vi "GetCurPageFromTabCtrl.vi"(11 "tab ctrl in":refnum<vi>) -> (2 "값":variant, 3 "tab ctrl out":refnum<vi>)   [LabVIEW 2018, in "Library-Ctrl.lvlib"]
uses:
  Library-Ctrl.lvlib
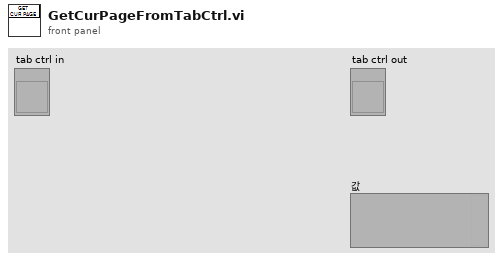
[diagram p1: front panel]
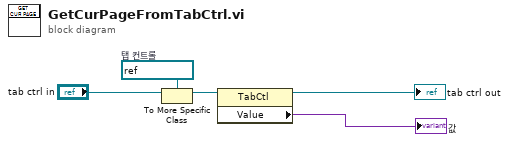
[diagram p0: block diagram]
diagram:
  w4 = refnum<vi> refnum  # 탭 컨트롤
  n1 = To More Specific Class(target class=w4, reference="tab ctrl in") -> (specific class reference=w3:refnum<vi>)  [unwired: 1 in, 1 out]
  n2 = property class="TabCtl"(reference=w3) -> (reference out=→"tab ctrl out":refnum<vi>, "Value"=→"값":variant)  [unwired: 1 in, 1 out]
